vi "Agilent 3446X Series Acquire Single.vi"() -> ()   [LabVIEW 2013]
doc: "This example shows how to configure a measurement and take a reading."
uses:
  <instrlib>/Agilent 3446X Series/Public/Data/Read (Single Point).vi
  <instrlib>/Agilent 3446X Series/Agilent 3446X Series.lvlib
panel:
  in  "Measurement Function (10: Voltage DC)":i32(ring)=10 items=["Continuity", "Current AC", "Current DC", "Diode", "Frequency", "Resistance 4-wire", "Period", "Resistance 2-wire", "Temperature", "Voltage AC", "Voltage DC", "Voltage DC Ratio", "Capacitance"]
  in  "Absolute Resolution (1E-6)":dbl=1e-06
  in  "VISA resource name":refnum<visa-resource-name>
  in  "Manual Range (1)":dbl=1.0
  in  "Auto Range (T: Enable)":bool=TRUE
  out "Measurement":dbl
  # "(c) 2013-2021 National Instruments.  ALL RIGHTS RESERVED."
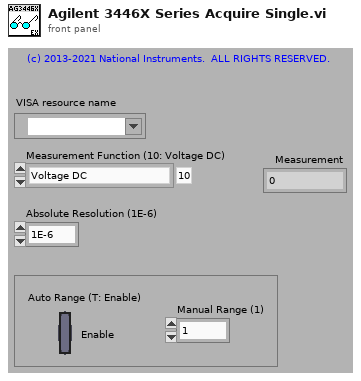
[diagram p1: front panel]
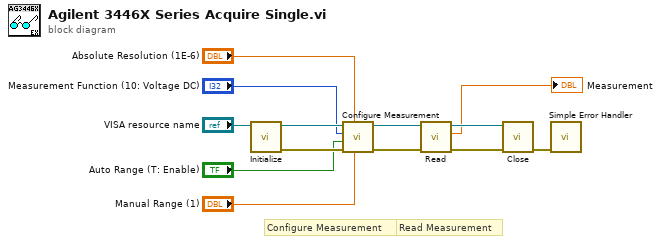
[diagram p0: block diagram]
diagram:
  # "Read Measurement"
  # "Configure Measurement"
  n1 = call <instrlib>:"Initialize.vi"("VISA resource name"="VISA resource name") -> ("error out"=w11:errorcluster, "VISA resource name out"=w12:refnum<visa-resource-name>)  [unwired: 4 in, 5 out]
  n2 = call <instrlib>:"Configure Measurement.vi"("Manual Range (1)"="Manual Range (1)", "Absolute Resolution (1E-6)"="Absolute Resolution (1E-6)", "error in (no error)"=w11, "Auto Range (T: Enable)"="Auto Range (T: Enable)", "Measurement Function (10: Voltage DC)"="Measurement Function (10: Voltage DC)", "VISA resource name"=w12) -> ("error out"=w7:errorcluster, "VISA resource name out"=w8:refnum<visa-resource-name>)  [unwired: 4 out]
  n3 = call-poly <instrlib>:"Read.vi"("error in (no error)"=w7, "VISA resource name"=w8) -> ("error out"=w10:errorcluster, "Measurement"=→"Measurement":dbl, "VISA resource name out"=w9:refnum<visa-resource-name>)  [unwired: 7 out]
  n4 = call <instrlib>:"Close.vi"("error in (no error)"=w10, "VISA resource name"=w9) -> ("error out"=w13:errorcluster)  [unwired: 9 out]
  n5 = call <vilib>:"Simple Error Handler.vi"("error in (no error)"=w13) -> ()  [unwired: 1 in, 8 out]
